vi "load_testprofile_parameters2.vi"(7 "error in (no error)":errorcluster, 9 "path":path=path "C:/Users/christian.acosta/Documents/Projects dev/Stations/Dependencies/TestProfile_OP60_GreyWall_Rev2p3.csv", 10 "index (row)":i32) -> (0 "error out":errorcluster, 2 "subarray":dbl[](array[numeric]), 3 "array count":i32)   [LabVIEW 2018]
uses:
  SupportVIs/Read Delimited Spreadsheet (string).vi
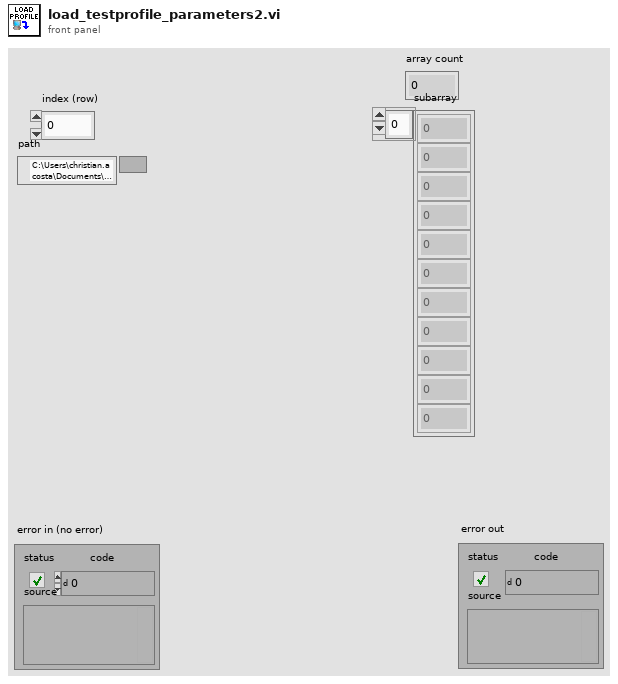
[diagram p1: front panel]
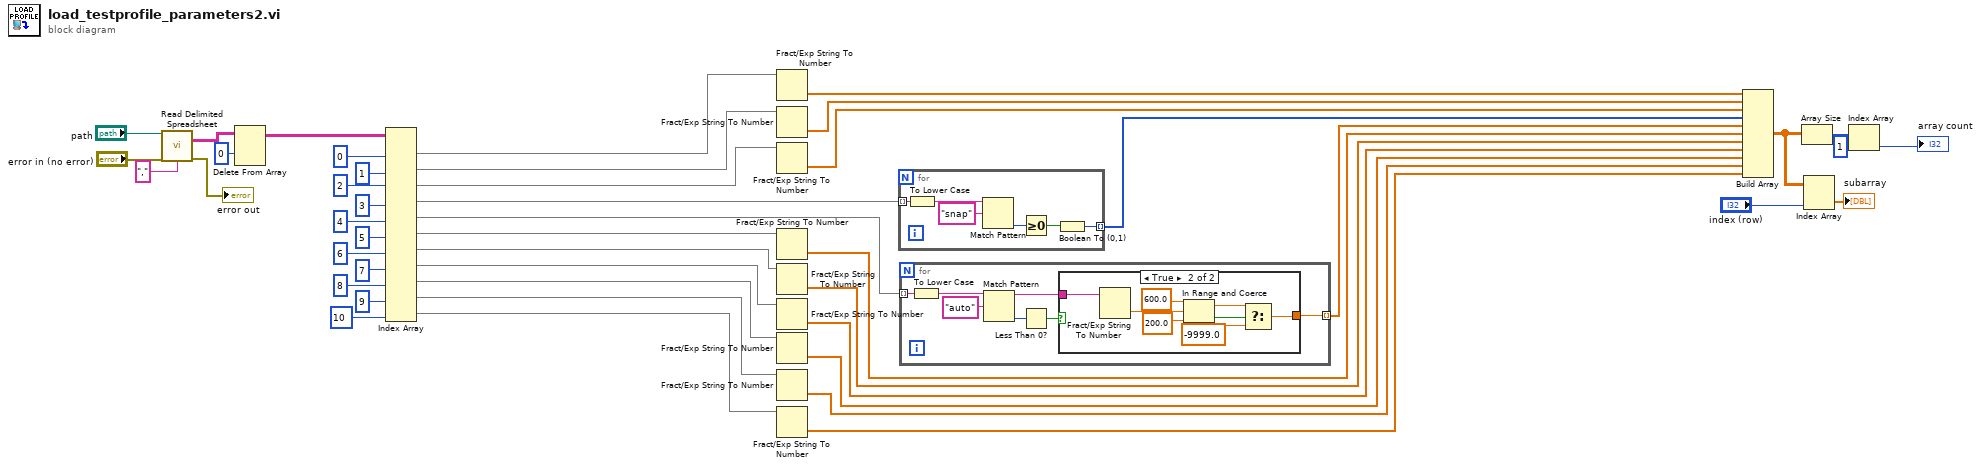
[diagram p0: block diagram]
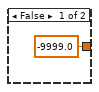
[diagram p2: hidden frame]
diagram:
  n1 = call-poly "Read Delimited Spreadsheet.vi"("file path (dialog if empty)"="path", "error in (no error)"="error in (no error)", "delimiter (\\t)"="," ("delimiter (\\t)")) -> ("all rows"=w44:string[][], "error out"=→"error out":errorcluster)  [unwired: 7 in, 4 out]
  n2 = Delete From Array(array=w44, index (row)=0) -> (array with subset deleted=w42:string[][])  [unwired: 2 in, 1 out]
  n3 = Index Array(array=w42, index (col) #1=0 ("disabled index (col)"), index (col) #2=1 ("disabled index (col)"), index (col) #3=2 ("disabled index (col)"), index (col) #4=3 ("disabled index (col)"), index (col) #5=4 ("disabled index (col)"), index (col) #6=5 ("disabled index (col)"), index (col) #7=6 ("disabled index (col)"), index (col) #8=7 ("disabled index (col)"), index (col) #9=8 ("disabled index (col)"), index (col) #10=9 ("disabled index (col)"), index (col) #11=10 ("index (col)")) -> (element #1=w40:string[], element #2=w39:string[], element #3=w38:string[], element #4=w37:string[], element #5=w36:string[], element #6=w35:string[], element #7=w34:string[], element #8=w33:string[], element #9=w32:string[], element #10=w31:string[], element #11=w6:string[])  [unwired: 11 in]
  n4 = Fract/Exp String To Number(string=w40) -> (number=w30:dbl[])  [unwired: 3 in, 1 out]
  n5 = Fract/Exp String To Number(string=w39) -> (number=w29:dbl[])  [unwired: 3 in, 1 out]
  n6 = Fract/Exp String To Number(string=w38) -> (number=w28:dbl[])  [unwired: 3 in, 1 out]
  n7 = Fract/Exp String To Number(string=w35) -> (number=w25:dbl[])  [unwired: 3 in, 1 out]
  n8 = Fract/Exp String To Number(string=w34) -> (number=w24:dbl[])  [unwired: 3 in, 1 out]
  n9 = Fract/Exp String To Number(string=w33) -> (number=w23:dbl[])  [unwired: 3 in, 1 out]
  n10 = Fract/Exp String To Number(string=w32) -> (number=w22:dbl[])  [unwired: 3 in, 1 out]
  n11 = Fract/Exp String To Number(string=w31) -> (number=w21:dbl[])  [unwired: 3 in, 1 out]
  n12 = Fract/Exp String To Number(string=w6) -> (number=w5:dbl[])  [unwired: 3 in, 1 out]
  n13 = for {
    tunnel: w37 -> [w52] mode=indexing
    tunnel: [w47] -> w27 mode=indexing
    n14 = To Lower Case(string=w52) -> (all lower case string=w51:string)
    n15 = Match Pattern(string=w51, regular expression="snap") -> (offset past match=w49:i32)  [unwired: 1 in, 3 out]
    n16 = Greater Or Equal To 0?(x=w49) -> (x >= 0?=w48:bool)
    n17 = Boolean To (0,1)(Boolean=w48) -> (0, 1=w47:i16)
  }
  n18 = for {
    tunnel: w36 -> [w59] mode=indexing
    tunnel: [w53] -> w26 mode=indexing
    n19 = To Lower Case(string=w59) -> (all lower case string=w58:string)
    n20 = Match Pattern(string=w58, regular expression="auto") -> (before substring=w54:string, offset past match=w56:i32)  [unwired: 1 in, 2 out]
    n21 = Less Than 0?(x=w56) -> (x < 0?=w55:bool)
    n22 = case shown="True" w55 {
      tunnel: w54 -> [_ w65]
      tunnel: [-9999.0 ("lower limit") w62] -> w53
      frame False {
      }
      frame True {
        n23 = Fract/Exp String To Number(string=w65) -> (number=w68:dbl)  [unwired: 3 in, 1 out]
        n24 = In Range and Coerce(upper limit=600.0, x=w68, lower limit=200.0) -> (coerced(x)=w63:dbl, In Range?=w64:bool)
        n25 = Select(t=w63, s=w64, f=-9999.0 ("lower limit")) -> (s? t:f=w62:dbl)
      }
    }
  }
  n26 = Build Array(w30, w29, w28, w27, w26, w25, w24, w23, w22, w21, w5) -> (w4:dbl[][])
  n27 = Array Size(array=w4) -> (size(s)=w8:i32[])
  n28 = Index Array(array=w4, index (col)="index (row)") -> (element=→"subarray":dbl[])  [unwired: 1 in]
  n29 = Index Array(array=w8, index=1) -> (element=→"array count":i32)
